vi "TypeCPRNum(SubVI).vi"() -> (0 "CprOut":string, 1 "Boolean":bool=TRUE)   [LabVIEW 2013, in "main.lvlib"]
uses:
  main.lvlib
  Controls/Enum Variables.ctl
  <vilib>/regexp/Match Regular Expression.xnode
panel:
  out "PatientID_TitleString":string
  in  "PatientID_ClearBtn":bool caption="ClearBtn"
  out "warning (transparent)":string="Der skal være 10 tal i et CPR nr"
  in  "PatientID_CancelBtn1":bool caption="CancelBtn1"
  in  "PatientID_OkBtn":bool caption="OkBtn"
  in  "PatientID_CPR Number Str":string caption="Patient ID"
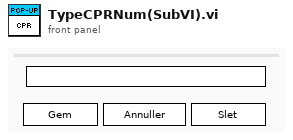
[diagram p1: front panel]
types:
  T1 = typedef "main.lvlib/Enum Variables.ctl" = enum16{"SetAcqFilter", "GetAcqFilter", "Set Filter", "Get Filter", "Set Height", "Get Height", "Set Recorded Height", "Get Recorded Height", "Set Blue Pressure", "Get Blue Pressure", "Set Red Pressure", "Get Red Pressure", "Init", "Reset Pressure", "Set Red Cursors", "Get Red Cursors", "Set Blue Cursors", "Get Blue Cursors", "Set Language", "Get Language", "Set Active Graphs", "Get ActiveGraphs", "Set Method", "Get Method", "Set Encryption", "Get Encryption", "Set ExcelVersion", "Get ExcelVersion", "Set DICOM Avail", "Get DICOM Avail", "Set DICOM Encode", "Get DICOM Encode", "Set JournalExport", "Get JournalExport", "Set Sequence", "Get Sequence", "Set DAQ Connected", "Get DAQ Connected", "Set Current Graph", "Get Current Graph", "Set General Settings", "Get Hyphenation", "Set Arm Calc Method", "Get Arm Calc Method", "Set Dicom Tags", "Get Dicom Tags", "Set BT Serial", "Get BT Serial", "Set BT Accepted Serials", "Get BT Accepted Serials", "Get BT License", "Set BT License"}
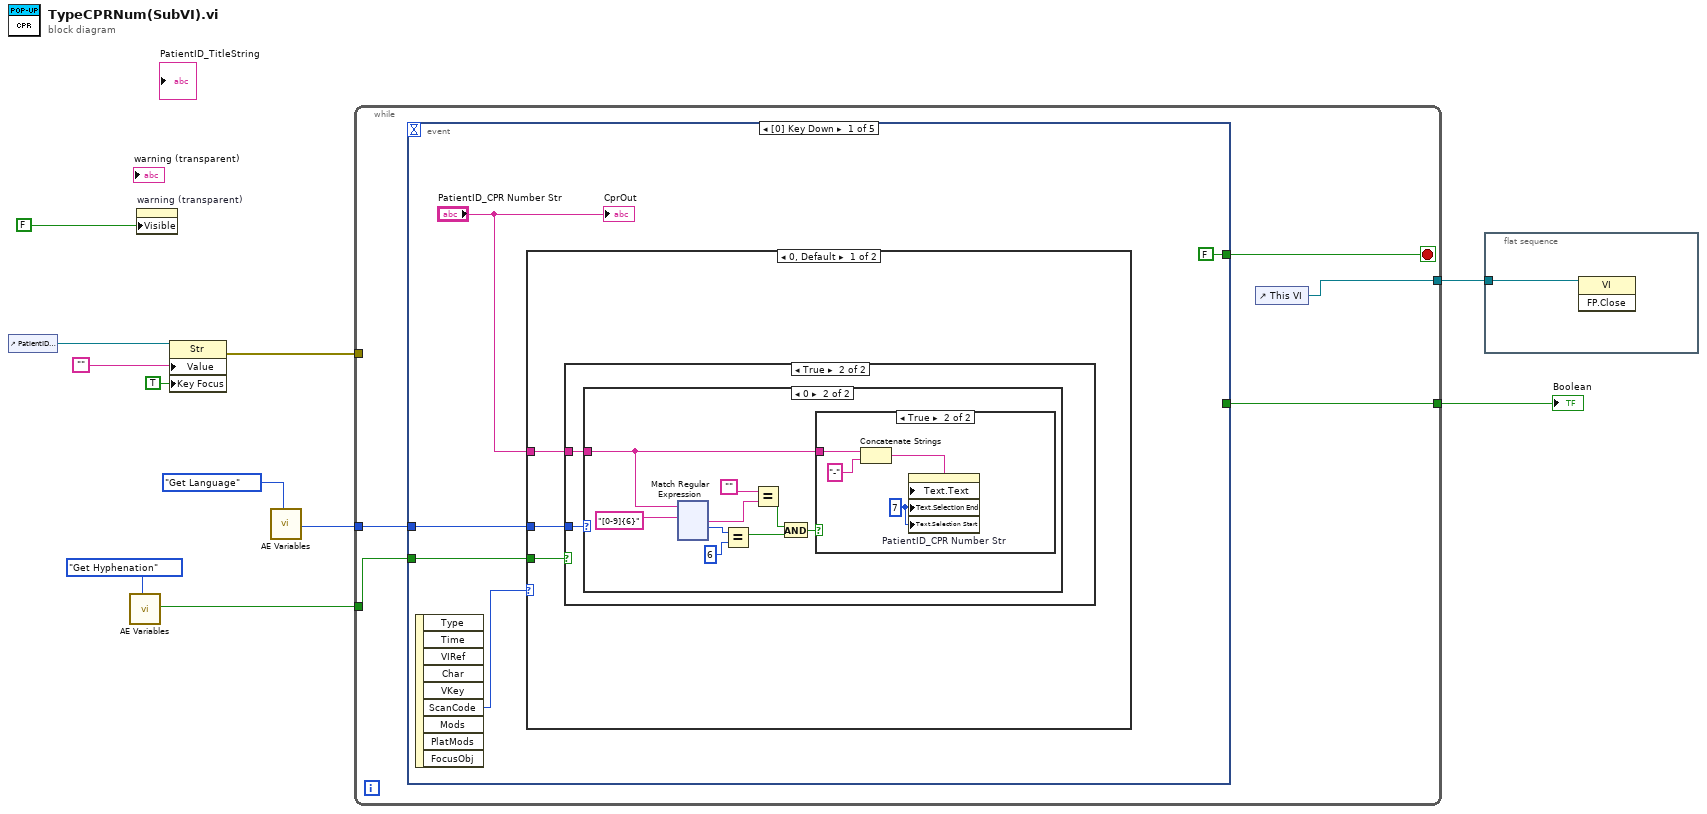
[diagram p0: block diagram]
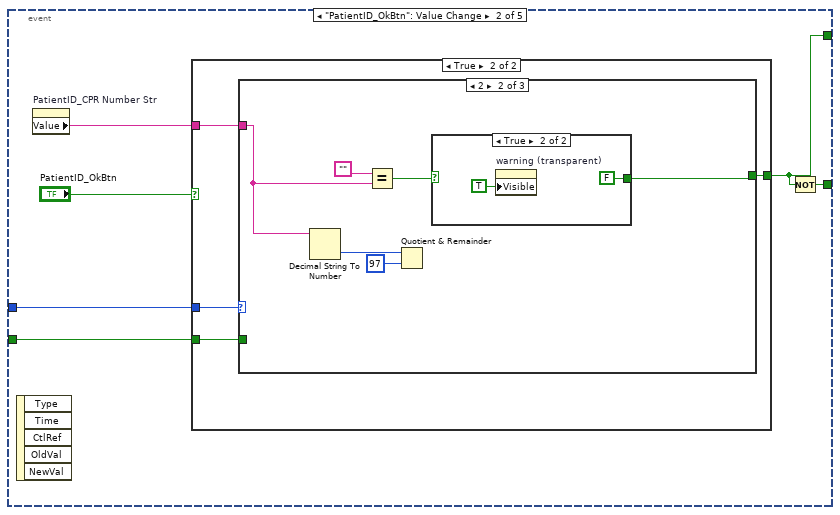
[diagram p6: hidden frame]
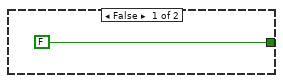
[diagram p7: hidden frame]
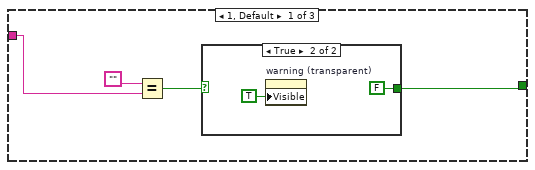
[diagram p8: hidden frame]
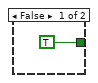
[diagram p9: hidden frame]
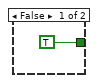
[diagram p10: hidden frame]
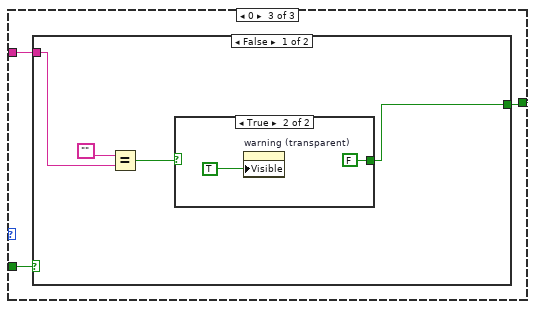
[diagram p11: hidden frame]
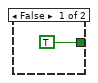
[diagram p12: hidden frame]
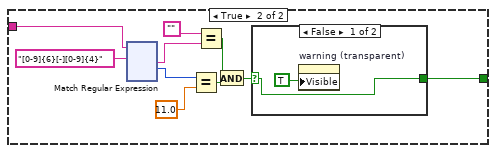
[diagram p13: hidden frame]
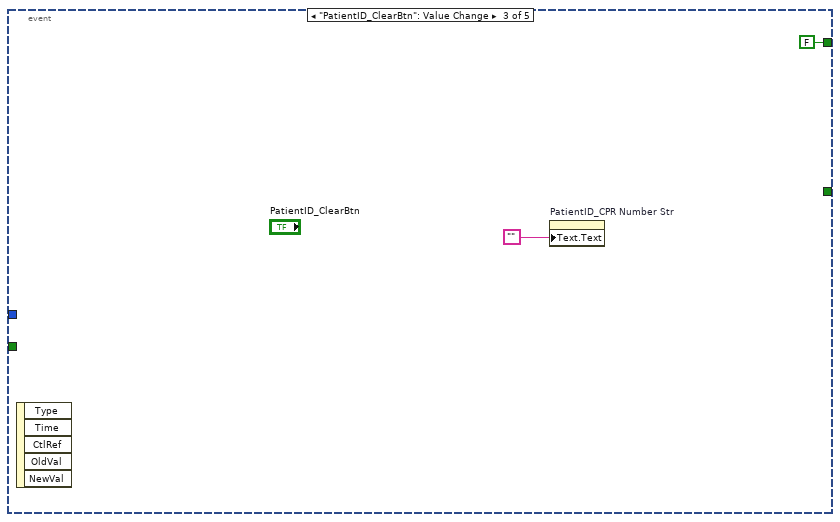
[diagram p15: hidden frame]
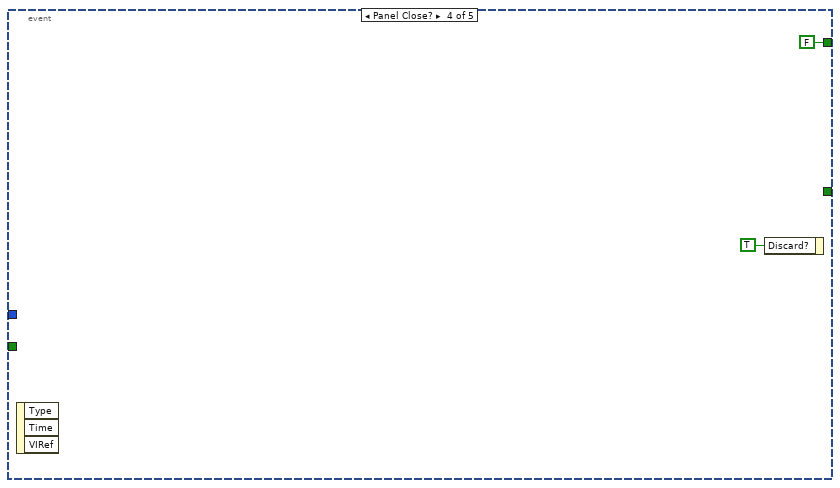
[diagram p16: hidden frame]
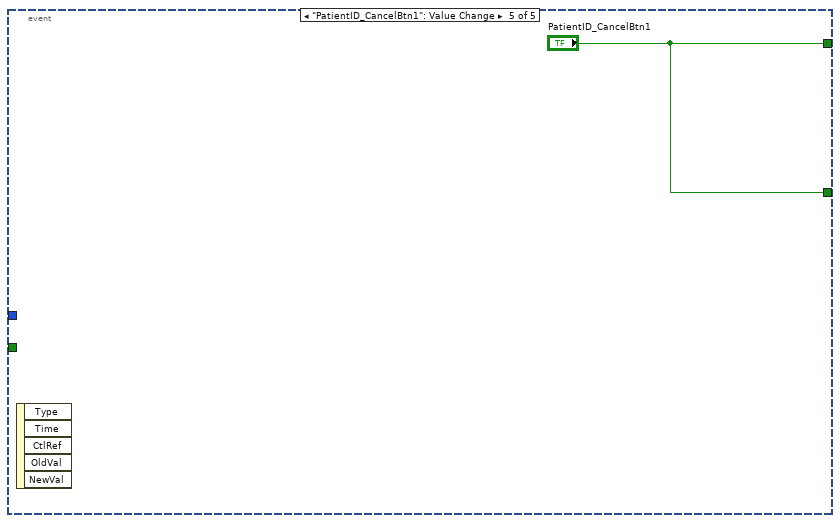
[diagram p17: hidden frame]
diagram:
  n1 = control-ref of="PatientID_CPR Number Str"() -> (w9:refnum<vi>)
  n2 = call "AE Variables.vi"("Action"=Enum_Variables."Get Hyphenation") -> ("BooleanOut"=w1:bool)  [unwired: 11 in, 7 out]
  n3 = property on="warning (transparent)" class="Str"("Visible"=FALSE) -> ()  [unwired: 2 in, 2 out]
  n4 = property class="Str"(reference=w9, "Value"="", "Key Focus"=TRUE) -> (error out=w6:errorcluster)  [unwired: 1 in, 1 out]
  n5 = call "AE Variables.vi"("Action"=Enum_Variables."Get Language") -> ("RingOut"=w4:u16)  [unwired: 11 in, 7 out]
  n6 = while {
    tunnel: [w15] -> w11
    tunnel: w6 -> [_]
    tunnel: w4 -> [w14]
    tunnel: [w13] -> w3
    tunnel: w1 -> [w12]
    stop <- w16 stop-if-true
    n7 = event shown="[0] Key Down" {
      selector: _ -> [_ _ _ _ _]
      dyn-events: _ -> [_ _ _ _ _]
      timeout: _ -> [_ _ _ _ _]
      tunnel: [FALSE ("CancelBtn1") w151 FALSE ("CancelBtn1") FALSE ("CancelBtn1") "PatientID_CancelBtn1"] -> w16
      tunnel: w14 -> [w18 w154 _ _ _]
      tunnel: [_ w153 _ _ "PatientID_CancelBtn1"] -> w13
      tunnel: w12 -> [w17 w152 _ _ _]
      event Key Down {
        n8 = event-data() -> ("ScanCode"=w20:i16)  [unwired: 1 in, 8 out]
        n9 = case shown="0, Default" w20 {
          tunnel: "PatientID_CPR Number Str" -> [w24 _]
          tunnel: w18 -> [w23 _]
          tunnel: w17 -> [w22 _]
          frame 0, Default {
            n10 = case shown="True" w22 {
              tunnel: w24 -> [_ w26]
              tunnel: w23 -> [_ w25]
              frame False {
              }
              frame True {
                n11 = case shown="0" w25 {
                  tunnel: w26 -> [_ w27]
                  frame Default {
                  }
                  frame 0 {
                    n12 = xnode "Match Regular Expression"("input string"=w27, "regular expression"="[0-9]{6}") -> ("after match"=w31:string, "offset past match"=w33:i32)  [unwired: 4 in, 3 out]
                    n13 = Equal?(x=w33, y=6) -> (x = y?=w30:bool)
                    n14 = Equal?(x="", y=w31) -> (x = y?=w29:bool)
                    n15 = And(x=w29, y=w30) -> (x .and. y?=w28:bool)
                    n16 = case shown="True" w28 {
                      tunnel: w27 -> [_ w150]
                      frame False {
                      }
                      frame True {
                        w147 = u32 7 ("Text.Selection:End")
                        n17 = Concatenate Strings(w150, "-" ("string")) -> (w148:string)
                        n18 = property on="PatientID_CPR Number Str" class="Str"("Text.Text"=w148, "Text.Selection End"=w147, "Text.Selection Start"=w147) -> ()  [unwired: 2 in, 2 out]
                      }
                    }
                  }
                }
              }
            }
          }
          frame 14 {
          }
        }
        "CprOut" <- "PatientID_CPR Number Str"
      }
      event "PatientID_OkBtn": Value Change {
        n19 = event-data() -> ()  [unwired: 1 in, 5 out]
        n20 = property on="PatientID_CPR Number Str" class="Str"() -> ("Value"=w155:string)  [unwired: 2 in, 2 out]
        n21 = case shown="True" "PatientID_OkBtn" {
          tunnel: w155 -> [_ w160]
          tunnel: [FALSE w161] -> w151
          tunnel: w154 -> [_ w159]
          tunnel: w152 -> [_ w158]
          frame False {
          }
          frame True {
            n22 = case shown="2" w159 {
              tunnel: [w163 w173 w180] -> w161
              tunnel: w160 -> [w164 w171 w179]
              tunnel: w158 -> [_ _ w178]
              frame 1, Default {
                n23 = Equal?(x="", y=w164) -> (x = y?=w162:bool)
                n24 = case shown="True" w162 {
                  tunnel: [TRUE FALSE] -> w163
                  frame False {
                  }
                  frame True {
                    n25 = property on="warning (transparent)" class="Str"("Visible"=TRUE) -> ()  [unwired: 2 in, 2 out]
                  }
                }
              }
              frame 2 {
                n26 = Decimal String To Number(string=w171) -> (number=w170:i32)  [unwired: 2 in, 1 out]
                n27 = Equal?(x="", y=w171) -> (x = y?=w172:bool)
                n28 = Quotient & Remainder(x=w170, y=97) -> ()  [unwired: 2 out]
                n29 = case shown="True" w172 {
                  tunnel: [TRUE FALSE] -> w173
                  frame False {
                  }
                  frame True {
                    n30 = property on="warning (transparent)" class="Str"("Visible"=TRUE) -> ()  [unwired: 2 in, 2 out]
                  }
                }
              }
              frame 0 {
                n31 = case shown="False" w178 {
                  tunnel: [w181 w197] -> w180
                  tunnel: w179 -> [w182 w193]
                  frame False {
                    n32 = Equal?(x="", y=w182) -> (x = y?=w183:bool)
                    n33 = case shown="True" w183 {
                      tunnel: [TRUE FALSE] -> w181
                      frame False {
                      }
                      frame True {
                        n34 = property on="warning (transparent)" class="Str"("Visible"=TRUE) -> ()  [unwired: 2 in, 2 out]
                      }
                    }
                  }
                  frame True {
                    n35 = xnode "Match Regular Expression"("input string"=w193, "regular expression"="[0-9]{6}[-][0-9]{4}") -> ("after match"=w191:string, "offset past match"=w194:i32)  [unwired: 4 in, 3 out]
                    n36 = Equal?(x=w194, y=11.0) -> (x = y?=w188:bool)
                    n37 = Equal?(x="", y=w191) -> (x = y?=w189:bool)
                    n38 = And(x=w189, y=w188) -> (x .and. y?=w190:bool)
                    n39 = case shown="False" w190 {
                      selector: w190 -> [w309 w311]
                      tunnel: [w309 w311] -> w197
                      frame False {
                        n40 = property on="warning (transparent)" class="Str"("Visible"=TRUE) -> ()  [unwired: 2 in, 2 out]
                      }
                      frame True {
                      }
                    }
                  }
                }
              }
            }
          }
        }
        n41 = Not(x=w151) -> (.not. x?=w153:bool)
      }
      event "PatientID_ClearBtn": Value Change {
        n42 = event-data() -> ()  [unwired: 1 in, 5 out]
        n43 = property on="PatientID_CPR Number Str" class="Str"("Text.Text"="") -> ()  [unwired: 2 in, 2 out]
      }
      event Panel Close? {
        n44 = event-data() -> ()  [unwired: 1 in, 3 out]
        n45 = event-data("Discard?"=TRUE) -> ()  [unwired: 1 in, 1 out]
      }
      event "PatientID_CancelBtn1": Value Change {
        n46 = event-data() -> ()  [unwired: 1 in, 5 out]
      }
    }
    n47 = control-ref of="This VI"() -> (w15:refnum<vi>)
  }
  "Boolean" <- w3
  n48 = flat-sequence {
    tunnel: w11 -> [w317]
    frame #0 {
      n49 = invoke class="VI" method="FP.Close"(reference=w317) -> ()  [unwired: 2 in, 3 out]
    }
  }
